vi "FG-Triggermode.vi"(8 "error in":errorcluster, 9 "Acquis. params. ref.":refnum<data-value>, 10 "Config file string in":string, 11 "Config. params. ref. in":refnum<data-value>) -> (0 "error IO":errorcluster, 1 "Number of replacements":i32, 2 "Config file string":string, 3 "Config. params. ref.":refnum<data-value>)   [LabVIEW 2013, in "CameraVision.lvlib" / "CV-Configuration.lvclass"]
uses:
  CV-Configuration.lvclass
  Acquisition/CV-Acquisition.lvclass
  CV-Configuration.lvclass/CV-Configuration.ctl
  Acquisition/CV-Acquisition.lvclass/CV-Acquisition.ctl
  Read Framegrabber DLL file.vi
  Read BoardHandle.vi
  Read Camport array.vi
  Acquisition/Read Trigger mode.vi
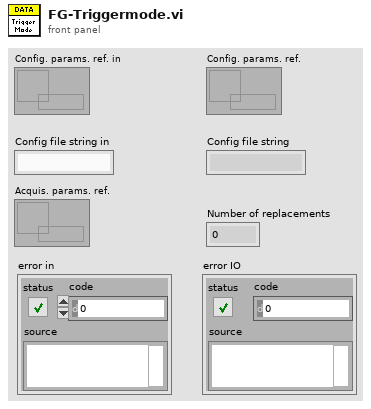
[diagram p1: front panel]
types:
  T1 = typedef "Trigger-modes.ctl" = enum16{"Camera timed (not sync.)", "Framegrabber timed (sync.)", "Software timed (sync.)", "External timing (sync.)", "Manual (sync.)", "Gated - camera (not sync.)", "Gated - grabber (sync.)", "Gated - software (sync.)", "Gated - external (sync.)"}
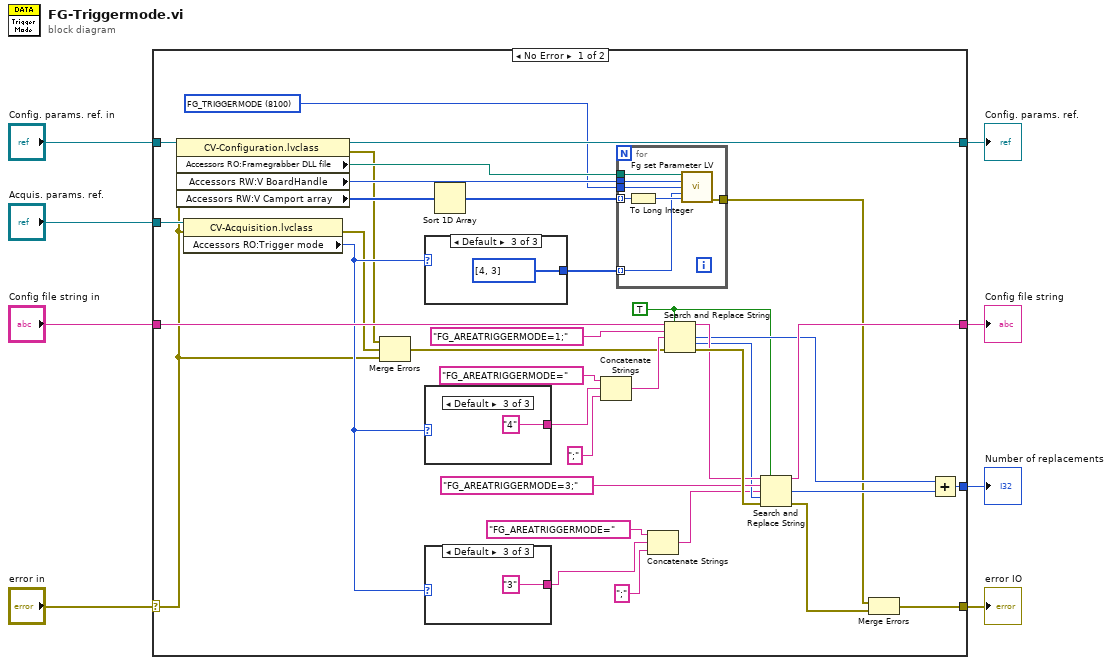
[diagram p0: block diagram]
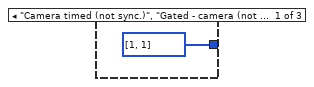
[diagram p2: hidden frame]
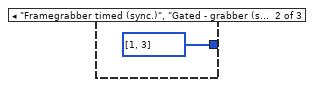
[diagram p3: hidden frame]
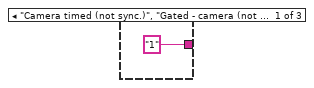
[diagram p4: hidden frame]
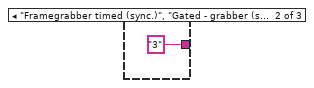
[diagram p5: hidden frame]
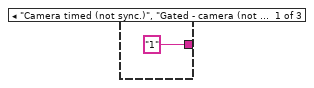
[diagram p6: hidden frame]
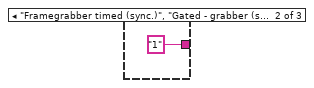
[diagram p7: hidden frame]
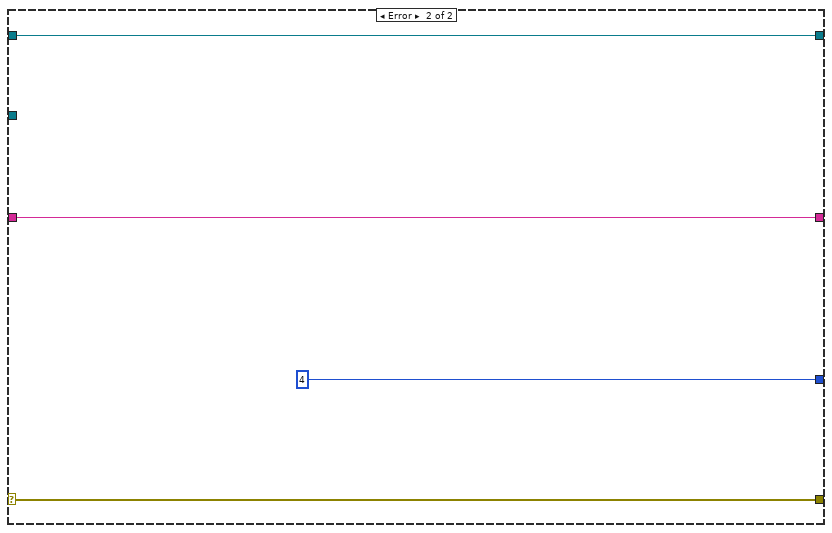
[diagram p8: hidden frame]
diagram:
  n1 = case shown="No Error" "error in" {
    selector: "error in" -> [w15 w63]
    tunnel: [w44 4] -> w8
    tunnel: [w11 w63] -> w7
    tunnel: [w42 w62] -> w6
    tunnel: "Config file string in" -> [w41 w62]
    tunnel: "Config. params. ref. in" -> [w24 w61]
    tunnel: "Acquis. params. ref." -> [w23 _]
    tunnel: [w22 w61] -> w1
    frame No Error {
      w19 = 8100 items=["FG_WIDTH"=100, "FG_HEIGHT"=200, "FG_FORMAT"=700, "FG_XOFFSET"=300, "FG_YOFFSET"=400, "FG_FRAMESPERSEC"=90, "FG_EXPOSURE"=10020, "FG_TRIGGERMODE"=8100, "FG_TRIGGERINSRC"=8110, "FG_CAMERA_LINK_CAMTYP"=11011, "FG_USEDVAL"=5025, "FG_SENSORREADOUT"=5050, "FG_STROBEPULSEDELAY"=8700, "FG_FLASH_POLARITY"=24060, "FG_EXSYNCINVERT"=8200, "FG_EXSYNCPOLARITY"=8420, "FG_EXSYNCDELAY"=8400, "FG_FLASHON"=8600, "FG_EXSYNCON"=8300, "FG_TRIGGERINPOLARITY"=8116, "FG_KNEE_LUT_FILE"=12110, "FG_KNEE_LUT_OFFSET"=12102, "FG_KNEE_LUT_SCALE"=12101, "FG_KNEE_LUT_GAMMA"=12103, "FG_KNEE_LUT_INVERT"=12104, "FG_CCSEL0"=14001, "FG_CCSEL1"=14002, "FG_CCSEL2"=14003, "FG_CCSEL3"=14004, "FG_DIGIO_OUTPUT"=14020, "FG_IMG_SELECT_PERIOD"=25110, "FG_IMG_SELECT"=25111, "FG_PORT"=3000, "FG_GLOBAL_ACCESS"=24110, "FG_TIMEOUT"=600] ("Ring")
      w25 = TRUE
      n2 = property class="CV-Configuration.lvclass"(reference=w24, error in=w15) -> (reference out=w22:refnum<data-value>, error out=w13:errorcluster, "Accessors RO:Framegrabber DLL file"=w21:path, "Accessors RW:V BoardHandle"=w20:u64, "Accessors RW:V Camport array"=w17:u32[])
      n3 = property class="CV-Acquisition.lvclass"(reference=w23, error in=w15) -> (error out=w12:errorcluster, "Accessors RO:Trigger mode"=w18:T1)  [unwired: 1 out]
      n4 = Merge Errors(w13, w12, w15) -> (w14:errorcluster)
      n5 = case shown="Default" w18 {
        tunnel: [u32[] [1, 1] u32[] [1, 3] u32[] [4, 3]] -> w16
        frame "Camera timed (not sync.)", "Gated - camera (not sync.)" {
        }
        frame "Framegrabber timed (sync.)", "Gated - grabber (sync.)" {
        }
        frame Default {
        }
      }
      n6 = case shown="Default" w18 {
        tunnel: ["1" "1" "4"] -> w27
        frame "Camera timed (not sync.)", "Gated - camera (not sync.)" {
        }
        frame "Framegrabber timed (sync.)", "Gated - grabber (sync.)" {
        }
        frame Default {
        }
      }
      n7 = case shown="Default" w18 {
        tunnel: ["1" "3" "3"] -> w26
        frame "Camera timed (not sync.)", "Gated - camera (not sync.)" {
        }
        frame "Framegrabber timed (sync.)", "Gated - grabber (sync.)" {
        }
        frame Default {
        }
      }
      n8 = Sort 1D Array(array=w17) -> (sorted array=w9:u32[])
      n9 = Concatenate Strings("FG_AREATRIGGERMODE=" ("string"), w27, ";" ("string")) -> (w37:string)
      n10 = for {
        tunnel: w21 -> [w51]
        tunnel: w20 -> [w50]
        tunnel: w19 -> [w49]
        tunnel: w9 -> [w48] mode=indexing
        tunnel: w16 -> [w46] mode=indexing
        tunnel: [w45] -> w10
        n11 = To Long Integer(number=w48) -> (32bit integer=w47:i32)
        n12 = call <userlib>:"Fg set Parameter LV.vi"("dll path in"=w51, "FgAddr"=w50, "Parameter"=w49, "Value"=w46, "CamPort"=w47) -> ("error out"=w45:errorcluster)  [unwired: 8 in, 2 out]
      }
      n13 = Concatenate Strings("FG_AREATRIGGERMODE=" ("string"), w26, ";" ("string")) -> (w28:string)
      n14 = Search and Replace String(replace all?=w25, input string=w41, search string="FG_AREATRIGGERMODE=1;", replace string=w37, error in=w14) -> (result string=w33:string, number of replacements=w32:i32, offset past replacement=w29:i32, error out=w34:errorcluster)  [unwired: 3 in]
      n15 = Search and Replace String(replace all?=w25, input string=w33, search string="FG_AREATRIGGERMODE=3;", replace string=w28, offset=w29, error in=w34) -> (result string=w42:string, number of replacements=w31:i32, error out=w43:errorcluster)  [unwired: 2 in, 1 out]
      n16 = Merge Errors(w10, w43) -> (w11:errorcluster)
      n17 = Add(x=w32, y=w31) -> (x+y=w44:i32)
    }
    frame Error {
    }
  }
  "Number of replacements" <- w8
  "error IO" <- w7
  "Config file string" <- w6
  "Config. params. ref." <- w1
